vi "Detect End of Injection.vi"(2 "Above Event Dwell Limit?":bool) -> (0 "Reset Event and Transition Counters?":bool)   [LabVIEW 2015]
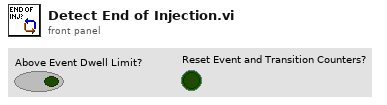
[diagram p1: front panel]
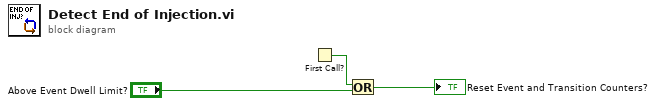
[diagram p0: block diagram]
diagram:
  n1 = First Call?() -> (First Call?: T/F=w3:bool)
  n2 = Or(x=w3, y="Above Event Dwell Limit?") -> (x .or. y?=→"Reset Event and Transition Counters?":bool)
